vi "ModelCheck_Rf.vi"(8 "error in (no error)":errorcluster, 11 "Data In":T1) -> (0 "error out":errorcluster, 3 "Data Out":T1)   [LabVIEW 2014]
uses:
  controls/Data.ctl
panel:
  # "日期"
  # "機種名稱"
  # "機種代號"
  # "商品條碼"
  # "台"
  # "OK"
  # "NG"
  # "台"
  # "總計"
  # "台"
  # "日期"
  # "機種名稱"
  # "機種代號"
  # "商品條碼"
  # "台"
  # "OK"
  # "NG"
  # "台"
  # "總計"
  # "台"
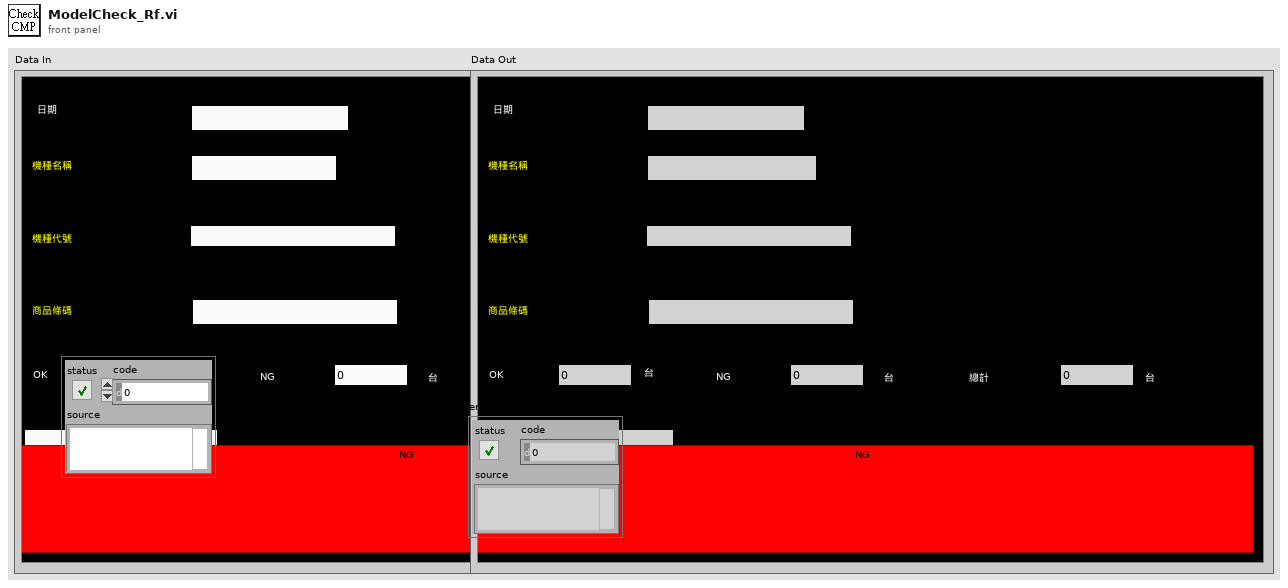
[diagram p1: front panel]
types:
  T1 = typedef "Data.ctl" = cluster{"Date":string, "BarCode1":string, "BarCode2":string, "BarCode3":string, "Message":string, "OK Count":u16, "NG Count":u16, "Total Count":u16, "ModelData":string[][], "OK&NG":bool, "COM1":refnum<visa-resource-name>, "COM2":refnum<visa-resource-name>, "IO":i32, "Time":u32, "TCP":refnum<k5>, "TCP 2":refnum<k5>}
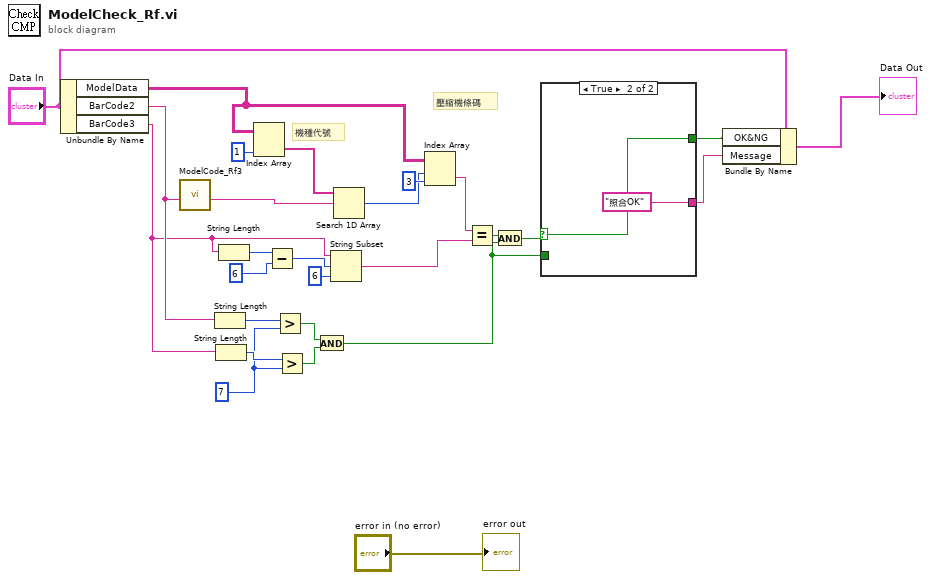
[diagram p0: block diagram]
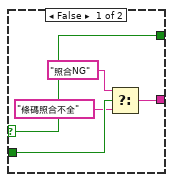
[diagram p2: hidden frame]
diagram:
  w12 = 7 ("y")
  # "壓縮機條碼"
  # "機種代號"
  n1 = Unbundle By Name("Data In") -> ("ModelData"=w18:string[][], "BarCode2"=w15:string, "BarCode3"=w2:string)
  n2 = call "ModelCode_Rf3.vi"("BarCode"=w15) -> ("ModeCode"=w16:string)  [unwired: 9 in, 1 out]
  n3 = String Length(string=w15) -> (length=w14:i32)
  n4 = String Length(string=w2) -> (length=w13:i32)
  n5 = String Length(string=w2) -> (length=w5:i32)
  n6 = Index Array(array=w18, index (col)=1 ("disabled index (col)")) -> (element=w26:string[])  [unwired: 1 in]
  n7 = Subtract(x=w5, y=6) -> (x-y=w3:i32)
  n8 = Greater?(x=w14, y=w12) -> (0:w11:bool)
  n9 = Greater?(x=w13, y=w12) -> (0:w10:bool)
  n10 = And(x=w11, y=w10) -> (x .and. y?=w7:bool)
  n11 = String Subset(string=w2, offset (0)=w3, length (rest)=6 ("length (rest)")) -> (substring=w1:string)
  n12 = Search 1D Array(1D array=w26, element=w16) -> (index of element=w24:i32)  [unwired: 1 in]
  n13 = Index Array(array=w18, index (row)=w24, index (col)=3 ("disabled index (col)")) -> (element=w17:string)
  n14 = Equal?(x=w17, y=w1) -> (x = y?=w9:bool)
  n15 = And(x=w9, y=w7) -> (x .and. y?=w8:bool)
  n16 = case shown="True" w8 {
    selector: w8 -> [w32 w34]
    tunnel: [w32 w34] -> w22
    tunnel: [w29 "照合OK" ("Message")] -> w19
    tunnel: w7 -> [w31 _]
    frame False {
      n17 = Select(t="照合NG" ("Message"), s=w31, f="條碼照合不全") -> (s? t:f=w29:string)
    }
    frame True {
    }
  }
  n18 = Bundle By Name(cluster="Data In", "OK&NG"=w22, "Message"=w19) -> (→"Data Out":T1)
  "error out" <- "error in (no error)"
